vi "offsetArrayIndex_every2.vi"(11 "y_offset_host array":fxp<+/-,16,8>[](array[numeric])) -> (3 "index":i32)   [LabVIEW 2017]
panel:
  out "size(s)":i32
  out "s? t:f":i32(graph)
  out "incr":i16(graph)
  out "count":u32
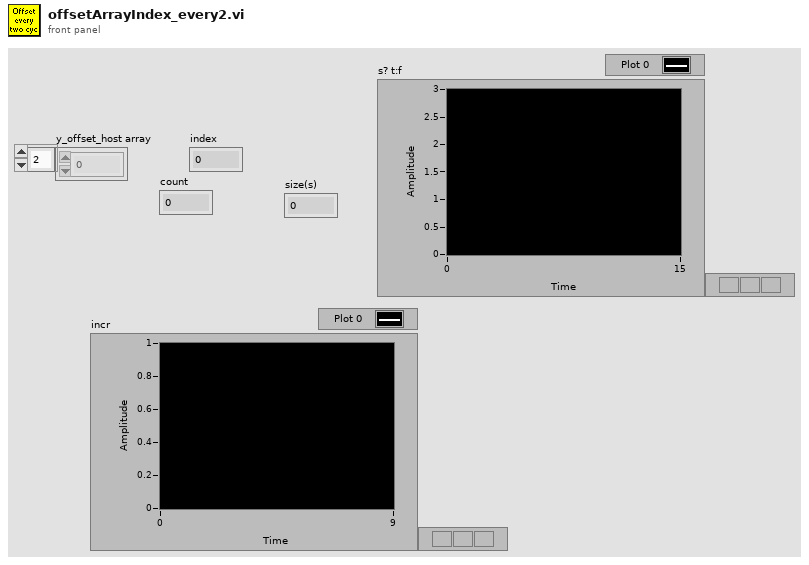
[diagram p1: front panel]
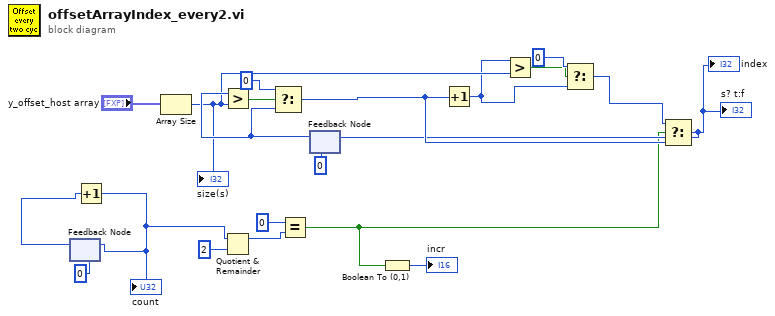
[diagram p0: block diagram]
diagram:
  n1 = feedback #1(u32 0 ("x")) -> (w14:u32)
  n2 = Increment(x=w14) -> (x+1=w13:u32)
  "count" <- w13
  n3 = feedback-in #1(w13) -> ()
  n4 = Array Size(array="y_offset_host array") -> (size(s)=w5:i32)
  "size(s)" <- w5
  n5 = Quotient & Remainder(x=w13, y=u32 2) -> (x-y*floor(x/y)=w11:u32)  [unwired: 1 out]
  n6 = Equal?(x=u32 0, y=w11) -> (x = y?=w7:bool)
  n7 = feedback #2(0 ("x")) -> (w16:i32)
  n8 = Greater?(x=w16, y=w5) -> (0:w18:bool)
  n9 = Select(t=0, s=w18, f=w16) -> (s? t:f=w9:i32)
  n10 = Boolean To (0,1)(Boolean=w7) -> (0, 1=→"incr":i16)
  n11 = Increment(x=w9) -> (x+1=w2:i32)
  n12 = Greater?(x=w2, y=w5) -> (0:w3:bool)
  n13 = Select(t=0, s=w3, f=w2) -> (s? t:f=w1:i32)
  n14 = Select(t=w1, s=w7, f=w9) -> (s? t:f=w8:i32)
  "index" <- w8
  "s? t:f" <- w8
  n15 = feedback-in #2(w8) -> ()
